vi "SetCol.vi"(4 "ModeCol Index":i32=2, 5 "Col Array Ref in":refnum<vi>, 6 "Cell Position":T1, 7 "Table History ref":refnum<vi>, 8 "error in (no error)":errorcluster, 9 "Table CtlRef In":refnum<vi>, 10 "SetTo":string, 11 "MenuDisableCol in":refnum<class "MenuDisableCol.lvclass">) -> (0 "error out":errorcluster, 1 "Table CtlRef Out":refnum<vi>, 2 "Num Rows":i32, 3 "MenuDisableCol out":refnum<class "MenuDisableCol.lvclass">)   [LabVIEW 2013, in "MenuDisableCol.lvclass"]
uses:
  MenuDisableCol.lvclass
  <vilib>/Utility/miscctls.llb/LVRowAndColumnTypeDef.ctl
  TypeDefs/TableHistory.ctl
  TypeDefs/TableArray.ctl
  MenuCol/MenuCol.lvclass
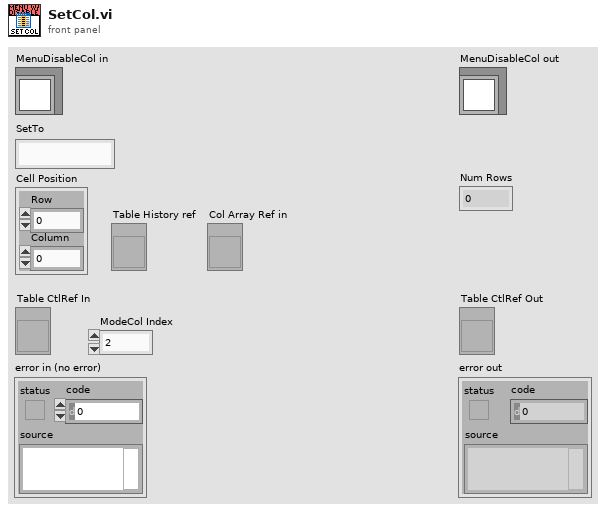
[diagram p1: front panel]
types:
  T1 = typedef "LVRowAndColumnTypeDef.ctl" = cluster{"Row":i32, "Column":i32}
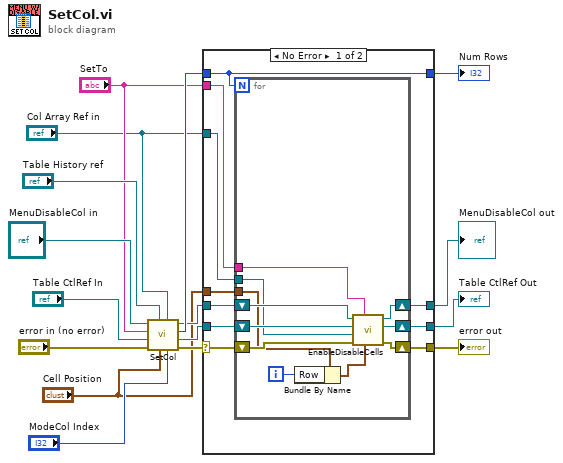
[diagram p0: block diagram]
diagram:
  n1 = call-parent "SetCol.vi"("ModeCol Index"="ModeCol Index", "Col Array Ref in"="Col Array Ref in", "Cell Position"="Cell Position", "Table History ref"="Table History ref", "error in (no error)"="error in (no error)", "Table CtlRef In"="Table CtlRef In", "SetTo"="SetTo", "MenuCol in"="MenuDisableCol in") -> ("error out"=w11:errorcluster, "Table CtlRef Out"=w9:refnum<vi>, "Num Rows"=w7:i32, "MenuCol out"=w5:refnum<class "MenuDisableCol.lvclass">)
  n2 = case shown="No Error" w11 {
    selector: w11 -> [w21 w41]
    tunnel: [w26 w41] -> w10
    tunnel: w9 -> [w20 w40]
    tunnel: [w25 w40] -> w8
    tunnel: w7 -> [w17 w39]
    tunnel: [w17 w39] -> w6
    tunnel: w5 -> [w22 w38]
    tunnel: [w24 w38] -> w4
    tunnel: "SetTo" -> [w23 _]
    tunnel: "Col Array Ref in" -> [w19 _]
    tunnel: "Cell Position" -> [w18 _]
    frame No Error {
      n3 = for {
        N: w17 -> [_]
        tunnel: w23 -> [w34]
        tunnel: w19 -> [w30]
        shift-right: [w35] -> w24
        shift-left: w22 -> [w33]
        shift-right: [w36] -> w25
        shift-left: w20 -> [w31]
        shift-right: [w37] -> w26
        shift-left: w21 -> [w32]
        tunnel: w18 -> [w29]
        i -> [w28]
        n4 = Bundle By Name(cluster=w29, "Row"=w28) -> (w27:T1)
        n5 = call-dynamic "EnableDisableCells.vi"("Cell Position"=w27, "Item Name or Tag"=w34, "error in (no error)"=w32, "Col Array Ref in"=w30, "Table CtlRef in"=w31, "MenuDisableCol in"=w33) -> ("error out"=w37:errorcluster, "Table CtlRef out"=w36:refnum<vi>, "MenuDisableCol out"=w35:refnum<class "MenuDisableCol.lvclass">)  [unwired: 2 in, 1 out]
      }
    }
    frame Error {
    }
  }
  "MenuDisableCol out" <- w4
  "Num Rows" <- w6
  "Table CtlRef Out" <- w8
  "error out" <- w10
